vi "DMCConfiguatorGui.FileWrite.vi"(8 "error in (no error)":errorcluster, 10 "ConfigData":T1[](array[typedef])) -> (0 "error out":errorcluster)   [LabVIEW 2016]
uses:
  DMCConfiguatorGui.ConfigData.ctl
  DMCConfiguatorGui.Component.ctl
  DMCConfiguatorGui.Type.ctl
  DMCConfiguatorGui.Var.ctl
  Global/ApplicationGlobal.vi
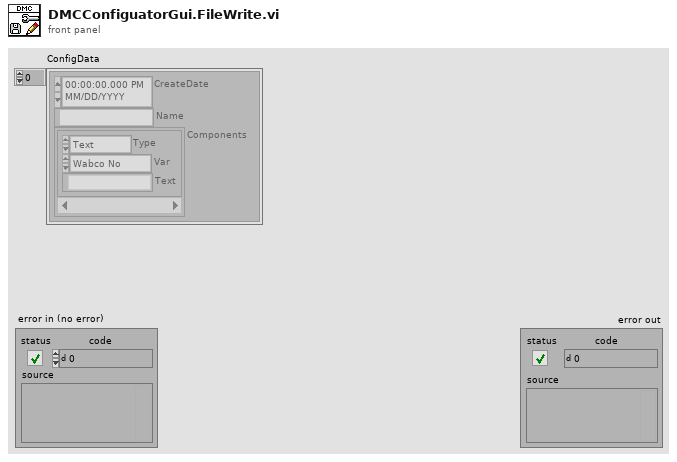
[diagram p1: front panel]
types:
  T1 = typedef "DMCConfiguatorGui.ConfigData.ctl" = cluster{"CreateDate":timestamp, "Name":string, "Components":T2[]}
  T2 = typedef "DMCConfiguatorGui.Component.ctl" = cluster{"Type":T3, "Var":T4, "Text":string}
  T3 = typedef "DMCConfiguatorGui.Type.ctl" = enum8{"Text", "Variable"}
  T4 = typedef "DMCConfiguatorGui.Var.ctl" = enum8{"-", "Wabco No", "Client No", "Serial", "Date"}
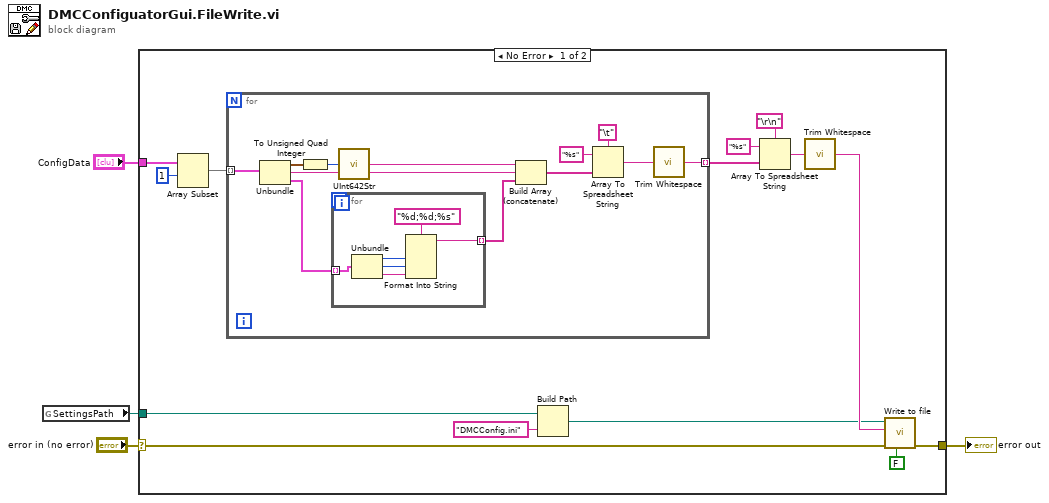
[diagram p0: block diagram]
diagram:
  n1 = global read "ApplicationGlobal.vi" "SettingsPath"() -> (w2:path)
  n2 = case shown="No Error" "error in (no error)" {
    selector: "error in (no error)" -> [w8 w37]
    tunnel: [w18 w37] -> w3
    tunnel: w2 -> [w17 _]
    tunnel: "ConfigData" -> [w7 _]
    frame No Error {
      n3 = Array Subset(array=w7, index=1) -> (w6:T1[])  [unwired: 1 in]
      n4 = for {
        tunnel: w6 -> [w30] mode=indexing
        tunnel: [w19] -> w13 mode=indexing
        n5 = Unbundle(w30) -> ("CreateDate"=w29:timestamp, "Name"=w26:string, "Components"=w25:T2[])
        n6 = To Unsigned Quad Integer(1:w29) -> (0:w28:u64)
        n7 = for {
          tunnel: w25 -> [w36] mode=indexing
          tunnel: [w31] -> w21 mode=indexing
          n8 = Unbundle(w36) -> ("Type"=w35:T3, "Var"=w34:T4, "Text"=w33:string)
          n9 = Format Into String(format string="%d;%d;%s", w35, w34, w33) -> (resulting string=w31:string)  [unwired: 2 in, 1 out]
        }
        n10 = call "UInt642Str.vi"("Numeric"=w28) -> ("string"=w27:string)
        n11 = Build Array (concatenate)(w27, w26, w21) -> (w22:string[])
        n12 = Array To Spreadsheet String(delimiter (Tab)="\t", array=w22, 3:"%s" ("format string")) -> (spreadsheet string=w20:string)
        n13 = call <vilib>:"Trim Whitespace.vi"("string"=w20) -> ("trimmed string"=w19:string)  [unwired: 1 in]
      }
      n14 = Build Path(base path=w17, name or relative path="DMCConfig.ini" ("format string")) -> (appended path=w9:path)
      n15 = Array To Spreadsheet String(delimiter (Tab)="\r\n", array=w13, 3:"%s" ("format string")) -> (spreadsheet string=w11:string)
      n16 = call <vilib>:"Trim Whitespace.vi"("string"=w11) -> ("trimmed string"=w10:string)  [unwired: 1 in]
      n17 = call "Write to file.vi"("append (F)"=FALSE, "error in"=w8, "addition"=w10, "file"=w9) -> ("error out"=w18:errorcluster)  [unwired: 7 in]
    }
    frame Error {
    }
  }
  "error out" <- w3
